vi "Configure Limit Test.vi"(6 "Limit Line Display (F: Disable)":bool, 7 "Limit Test (F: Disable)":bool, 8 "error in (no error)":errorcluster, 9 "Limit Fail Display (F: Disable)":bool, 10 "Channel (1)":i32=1, 11 "VISA resource name":refnum<visa-resource-name>) -> (0 "error out":errorcluster, 3 "VISA resource name out":refnum<visa-resource-name>)   [LabVIEW 2012, in "Tektronix TTR500 Series.lvlib"]
doc: "This VI configures limit test parameters."
uses:
  <instrlib>/Tektronix TTR500 Series/Tektronix TTR500 Series.lvlib
panel:
  # "Enable\n\nDisable"
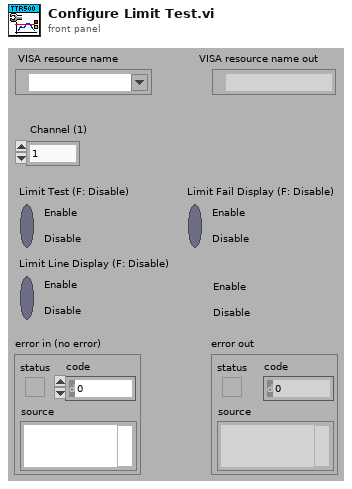
[diagram p1: front panel]
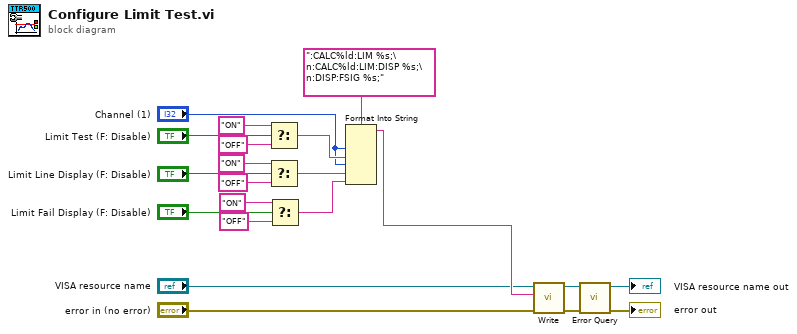
[diagram p0: block diagram]
diagram:
  n1 = Select(t="ON", s="Limit Test (F: Disable)", f="OFF") -> (s? t:f=w14:string)
  n2 = Select(t="ON", s="Limit Line Display (F: Disable)", f="OFF") -> (s? t:f=w13:string)
  n3 = Select(t="ON", s="Limit Fail Display (F: Disable)", f="OFF") -> (s? t:f=w9:string)
  n4 = Format Into String(format string=":CALC%ld:LIM %s;\n:CALC%ld:LIM:DISP %s;\n:DISP:FSIG %s;", "Channel (1)", w14, "Channel (1)", w13, w9) -> (resulting string=w3:string)  [unwired: 2 in, 1 out]
  n5 = call <instrlib>:"Write.vi"("error in (no error)"="error in (no error)", "String ()"=w3, "VISA resource name"="VISA resource name") -> ("error out"=w7:errorcluster, "VISA resource name out"=w8:refnum<visa-resource-name>)  [unwired: 6 in, 1 out]
  n6 = call <instrlib>:"Error Query.vi"("error in (no error)"=w7, "VISA resource name"=w8) -> ("error out"=→"error out":errorcluster, "VISA resource name out"=→"VISA resource name out":refnum<visa-resource-name>)  [unwired: 6 in, 2 out]
